vi "pp2_util_addToMean.vi"(8 "New value":dbl=7.0, 10 "Original count":i64=1, 11 "Original mean":dbl=3.0) -> (3 "New mean":dbl)   [LabVIEW 2013]
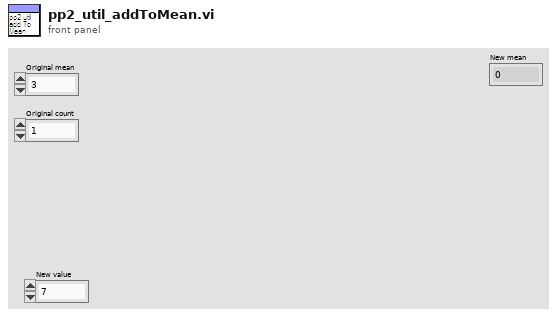
[diagram p1: front panel]
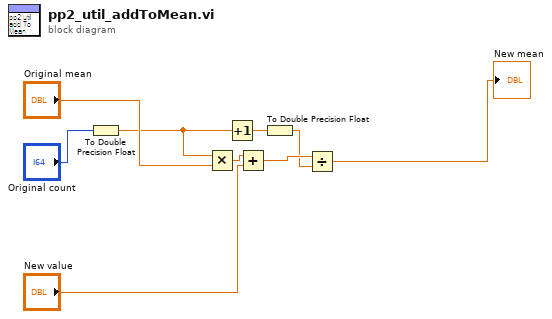
[diagram p0: block diagram]
diagram:
  n1 = To Double Precision Float(number="Original count") -> (double precision float=w1:dbl)
  n2 = Multiply(x=w1, y="Original mean") -> (x*y=w9:dbl)
  n3 = Increment(x=w1) -> (x+1=w4:dbl)
  n4 = Add(x=w9, y="New value") -> (x+y=w8:dbl)
  n5 = To Double Precision Float(number=w4) -> (double precision float=w3:dbl)
  n6 = Divide(x=w8, y=w3) -> (x/y=→"New mean":dbl)
